vi "2 HeadingChooser.vi"() -> (2 "Optimal Heading Out":dbl, 3 "Goodness Functions":T3, 10 "Goodness Weightings":T2={"Target Importance"=0.98, "No Sail Importance"=1.0, "Change Importance"=0.2, "Pure Waypoint \nImportance"=0.0, "Pure Wind \nImportance"=0.0} {"Pure Wind \nImportance" min=0.0 step=0.2; "Pure Waypoint \nImportance" min=0.0 step=0.2; "Change Importance" min=0.0 step=0.2; "No Sail Importance" min=0.0 step=0.2; "Target Importance" min=0.0 step=0.2})   [LabVIEW 2011]
doc: "The Heading Chooser VI is responsible for finding the optimal heading for the boat in order to reach the waypoint. It uses fuzzy-logic inspired goodness function logic to choose a heading. Specifically, the VI takes 3 goodness function curves and makes a weighted combination of them, choosing the heading with the highest total goodness.\n\nThis VI does not contain any code that would limit the component goodness functions to just 3 or to the specific ones of 'target', 'no sail', and 'change'. Only the labels would need changing."
uses:
  2 Typedefs/Goodness Fns Indicator.ctl
  2 Typedefs/Goodness Weightings.ctl
  2 Classes/Waypoint/Waypoint.lvclass
  2 Globals/2 TuningConstants.vi
  2 Globals/2 Global.vi
panel:
  in  "Irons direct vector":T1 {"Origin"."North" format="%#_10f"; "Origin"."East" format="%#_8f"}
  out "start of wire":dbl
  out "end of wire":dbl
  # "huh???\nTODO: talk to NI about this"
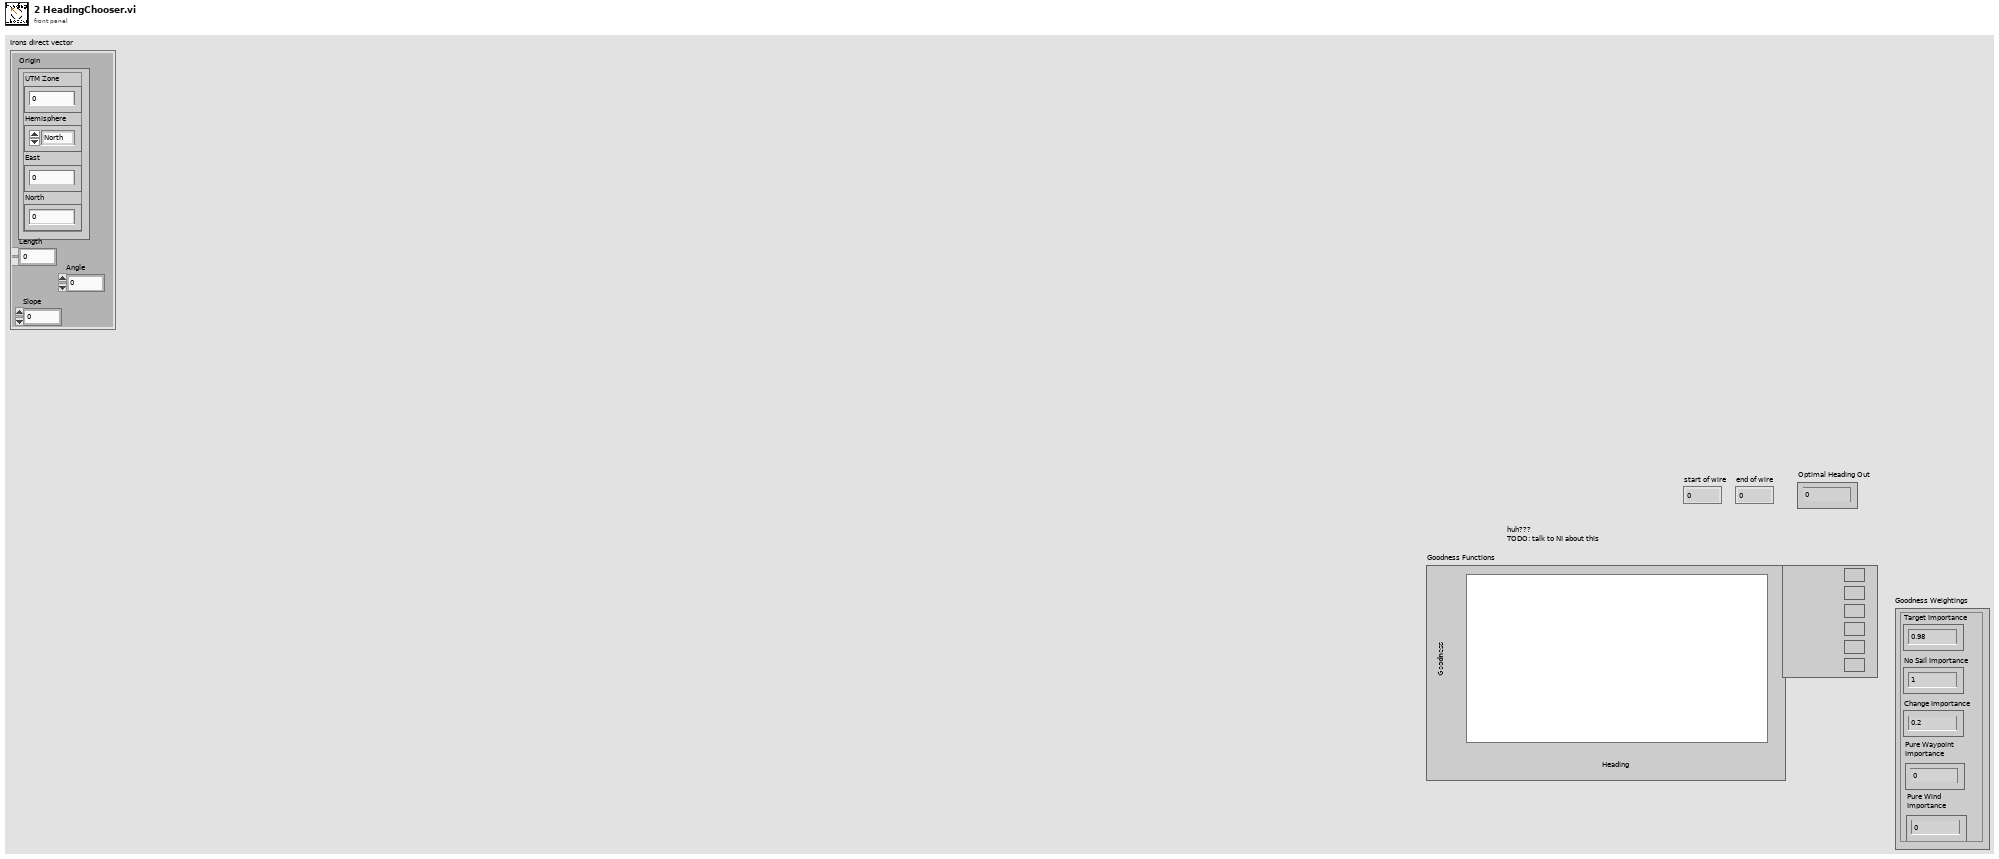
[diagram p1: front panel]
types:
  T1 = cluster{"Origin":cluster{"UTM Zone":dbl, "Hemisphere":enum16{"North", "South"}, "East":dbl, "North":dbl}, "Length":dbl, "Angle":dbl, "Slope":dbl}
  T2 = typedef "Goodness Weightings.ctl" = cluster{"Target Importance":dbl, "No Sail Importance":dbl, "Change Importance":dbl, "Pure Waypoint \nImportance":dbl, "Pure Wind \nImportance":dbl}
  T3 = typedef "Goodness Fns Indicator.ctl" = cluster{dbl, dbl, dbl[][]}
  T4 = typedef "UTM Location.ctl" = cluster{"UTM Zone":dbl, "Hemisphere":enum16{"North", "South"}, "East":dbl, "North":dbl}
  T5 = typedef "absolute wind direction.ctl" = dbl
  T6 = typedef "apparent wind direction.ctl" = dbl
  T7 = typedef "heading.ctl" = dbl
  T8 = cluster{"UTM Zone":dbl, "Hemisphere":enum16{"North", "South"}, "East":dbl, "North":dbl}
  T9 = cluster{"UTM Zone":bool, "Hemisphere":bool, "East":bool, "North":bool}
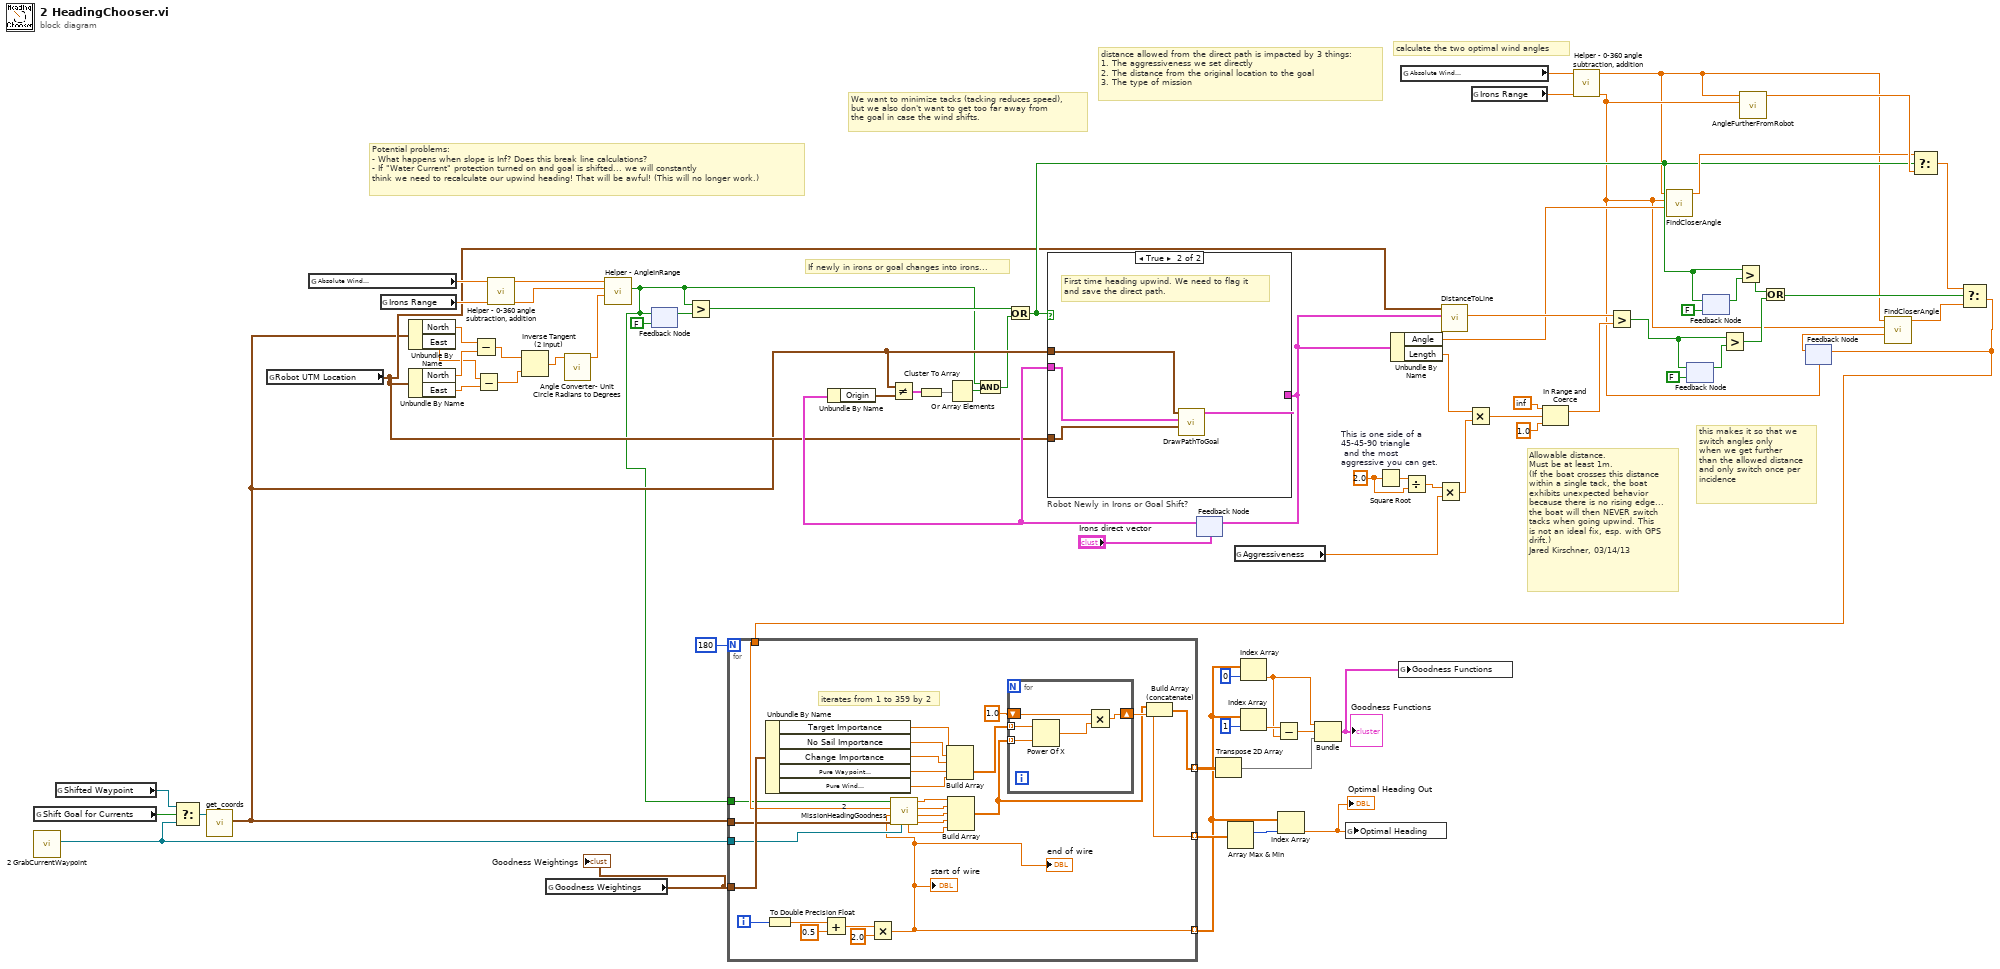
[diagram p0: block diagram]
diagram:
  w40 = 2.0 ("x")
  # "Potential problems:\n- What happens when slope is Inf? Does this break line calculations?\n- If \"Water Current\" protection turned on and goal is shifted... we will constantly\nthink we need to recalculate our upwind heading! That will be awful! (This will no longer work.)"
  # "If newly in irons or goal changes into irons..."
  # "Allowable distance.\nMust be at least 1m.\n(If the boat crosses this distance\nwithin a single tack, the boat\nexhibits unexpected behavior\nbecause there is no rising edge...\nthe boat will then NEVER switch\ntacks when going upwind. This\nis not an ideal fix, esp. with GPS\ndrift.)\nJared Kirschner, 03/14/13"
  # "this makes it so that we\nswitch angles only\nwhen we get further\nthan the allowed distance\nand only switch once per\nincidence"
  # "calculate the two optimal wind angles"
  # "distance allowed from the direct path is impacted by 3 things:\n1. The aggressiveness we set directly\n2. The distance from the original location to the goal\n3. The type of mission"
  # "We want to minimize tacks (tacking reduces speed),\nbut we also don't want to get too far away from\nthe goal in case the wind shifts."
  n1 = global read "2 Global.vi" "Shift Goal for Currents"() -> (w62:bool)
  n2 = call "2 GrabCurrentWaypoint.vi"() -> ("Current Waypoint"=w61:refnum<class "Waypoint.lvclass">)  [unwired: 11 in]
  n3 = global read "2 Global.vi" "Shifted Waypoint"() -> (w63:refnum<class "Waypoint.lvclass">)
  n4 = Select(t=w63, s=w62, f=w61) -> (s? t:f=w60:refnum<class "Waypoint.lvclass">)
  n5 = call-dynamic "get_coords.vi"("Waypoint in"=w60) -> ("Coords"=w17:T4)  [unwired: 7 in, 3 out]
  n6 = global read "2 Global.vi" "Robot UTM Location"() -> (w18:T4)
  n7 = global read "2 Global.vi" "Absolute Wind\nDirection (º)"() -> (w48:T5)
  n8 = global read "2 TuningConstants.vi" "Irons Range"() -> (w49:dbl)
  n9 = Unbundle By Name(w17) -> ("North"=w53:dbl, "East"=w51:dbl)
  n10 = Unbundle By Name(w18) -> ("North"=w52:dbl, "East"=w50:dbl)
  n11 = Subtract(x=w53, y=w52) -> (x-y=w56:dbl)
  n12 = Subtract(x=w51, y=w50) -> (x-y=w55:dbl)
  n13 = call "Helper - 0-360 angle subtraction, addition.vi"("y"=w49, "x"=w48) -> ("x + y"=w46:dbl, "x - y"=w47:T6)  [unwired: 8 in]
  n14 = Inverse Tangent (2 Input)(1:w55, 2:w56) -> (0:w54:dbl)
  n15 = global read "2 TuningConstants.vi" "Goodness Weightings"() -> (w69:T2)
  "Goodness Weightings" <- w69
  n16 = call "Angle Converter- Unit Circle Radians to Degrees.vi"("Angle in \nUnit Circle\nRadians"=w54) -> ("Angle in \nHeading \nFormat"=w57:T7)  [unwired: 10 in]
  n17 = call "Helper - AngleInRange.vi"("Angle to check"=w57, "Angle 2"=w46, "Angle 1"=w47) -> ("In range?"=w15:bool)  [unwired: 8 in]
  n18 = feedback-in #1(w15) -> ()
  n19 = feedback #1(FALSE ("In irons?")) -> (w44:bool)
  n20 = Greater?(x=w15, y=w44) -> (0:w28:bool)
  n21 = feedback #2("Irons direct vector") -> (w39:T1)
  n22 = Unbundle By Name(w39) -> ("Origin"=w38:T8)
  n23 = Not Equal?(x=w17, y=w38) -> (x != y?=w37:T9)
  n24 = Cluster To Array(cluster=w37) -> (array=w36:bool[])
  n25 = Or Array Elements(Boolean array=w36) -> (logical OR=w16:bool)
  n26 = And(x=w15, y=w16) -> (x .and. y?=w14:bool)
  n27 = Or(x=w28, y=w14) -> (x .or. y?=w20:bool)
  n28 = case "Robot Newly in Irons or Goal Shift?" shown="True" w20 {
    tunnel: w39 -> [w76 w80]
    tunnel: w17 -> [_ w79]
    tunnel: w18 -> [_ w78]
    tunnel: [w76 w77] -> w7
    frame False {
    }
    frame True {
      # "First time heading upwind. We need to flag it\nand save the direct path."
      n29 = call "DrawPathToGoal.vi"("Robot UTM Location"=w78, "Irons direct vector in"=w80, "Goal"=w79) -> ("Irons direct vector out"=w77:T1)  [unwired: 8 in]
    }
  }
  n30 = feedback-in #2(w7) -> ()
  n31 = global read "2 TuningConstants.vi" "Aggressiveness"() -> (w31:dbl)
  n32 = Square Root(x=w40) -> (sqrt(x)=w41:dbl)
  n33 = Unbundle By Name(w7) -> ("Angle"=w5:dbl, "Length"=w6:dbl)
  n34 = global read "2 Global.vi" "Absolute Wind\nDirection (º)"() -> (w34:T5)
  n35 = Divide "This is one side of a 45-45-90 triangle\n and the most aggressive you can get."(x=w41, y=w40) -> (x/y=w33:dbl)
  n36 = Multiply(x=w33, y=w31) -> (x*y=w32:dbl)
  n37 = call "DistanceToLine.vi"("Irons direct vector out"=w7, "Robot UTM Location"=w18) -> ("Distance"=w42:dbl)  [unwired: 9 in]
  n38 = Multiply(x=w6, y=w32) -> (x*y=w11:dbl)
  n39 = global read "2 TuningConstants.vi" "Irons Range"() -> (w35:dbl)
  n40 = In Range and Coerce(upper limit=inf, x=w11, lower limit=1.0) -> (coerced(x)=w10:dbl)  [unwired: 1 out]
  n41 = call "Helper - 0-360 angle subtraction, addition.vi"("y"=w35, "x"=w34) -> ("x + y"=w3:dbl, "x - y"=w2:T6)  [unwired: 8 in]
  n42 = Greater?(x=w42, y=w10) -> (0:w23:bool)
  n43 = call "FindCloserAngle.vi"("Central Angle"=w5, "Angle 2"=w3, "Angle 1"=w2) -> ("Closer Angle"=w26:T6)  [unwired: 8 in]
  n44 = feedback #3(FALSE) -> (w25:bool)
  n45 = feedback-in #3(w23) -> ()
  n46 = feedback #4(FALSE) -> (w21:bool)
  n47 = feedback-in #4(w20) -> ()
  n48 = Greater?(x=w23, y=w25) -> (0:w12:bool)
  n49 = Greater?(x=w20, y=w21) -> (0:w13:bool)
  n50 = call "AngleFurtherFromRobot.vi"("Angle 2"=w3, "Angle 1"=w2) -> ("Angle further from Robot"=w27:T6)  [unwired: 9 in]
  n51 = Or(x=w13, y=w12) -> (x .or. y?=w19:bool)
  n52 = feedback #5(w3) -> (w4:T6)
  n53 = call "FindCloserAngle.vi"("Central Angle"=w4, "Angle 2"=w3, "Angle 1"=w2) -> ("Closer Angle"=w1:T6)  [unwired: 8 in]
  n54 = Select(t=w26, s=w20, f=w27) -> (s? t:f=w30:T6)
  n55 = Select(t=w30, s=w19, f=w1) -> (s? t:f=w29:T6)
  n56 = for {
    N: 180 -> [_]
    tunnel: [w101] -> w67 mode=indexing
    tunnel: w69 -> [w105]
    tunnel: w61 -> [w104]
    tunnel: w17 -> [w103]
    tunnel: [w102] -> w68 mode=indexing
    tunnel: [w93] -> w59 mode=indexing
    tunnel: w29 -> [w82]
    tunnel: w15 -> [w81]
    i -> [w106]
    # "iterates from 1 to 359 by 2"
    n57 = Unbundle By Name(w105) -> ("Target Importance"=w88:dbl, "No Sail Importance"=w89:dbl, "Change Importance"=w90:dbl, "Pure Waypoint \nImportance"=w91:dbl, "Pure Wind \nImportance"=w92:dbl)
    n58 = To Double Precision Float(number=w106) -> (double precision float=w99:dbl)
    n59 = Add(x=w99, y=0.5) -> (x+y=w98:dbl)
    n60 = Multiply(x=w98, y=2.0) -> (x*y=w93:dbl)
    "end of wire" <- w93
    "start of wire" <- w93
    n61 = call "2 MissionHeadingGoodness.vi"("Waypoint in"=w104, "Waypoint Location"=w103, "Heading\nto Test"=w93, "UW Tack"=w82, "Into irons?"=w81) -> ("Pure Waypoint Goodness"=w84:dbl, "Direction Change Goodness"=w85:dbl, "No-Sail Goodness"=w86:dbl, "Target Goodness"=w87:dbl, "Pure Wind Goodness"=w83:dbl)  [unwired: 2 in]
    n62 = Build Array(w88, w89, w90, w91, w92) -> (w95:dbl[])
    n63 = Build Array(w87, w86, w85, w84, w83) -> (w94:dbl[])
    n64 = for {
      tunnel: w94 -> [w111] mode=indexing
      tunnel: w95 -> [w110] mode=indexing
      shift-right: [w108] -> w101
      shift-left: 1.0 -> [w107]
      n65 = Power Of X(1:w111, 2:w110) -> (0:w109:dbl)
      n66 = Multiply(x=w107, y=w109) -> (x*y=w108:dbl)
    }
    n67 = Build Array (concatenate)(w94, w101) -> (w102:dbl[])
  }
  n68 = Transpose 2D Array(2D array=w68) -> (transposed array=w64:dbl[][])
  n69 = Array Max & Min(array=w67) -> (max index (indices)=w71:i32)  [unwired: 3 out]
  n70 = Index Array(array=w59, index=0) -> (element=w66:dbl)
  n71 = Index Array(array=w59, index=1) -> (element=w74:dbl)
  n72 = Subtract(x=w74, y=w66) -> (x-y=w65:dbl)
  n73 = Index Array(array=w59, index=w71) -> (element=w58:dbl)
  "Optimal Heading Out" <- w58
  n74 = Bundle(w66, w65, w64) -> (w70:cluster{dbl, dbl, dbl[][]})  [unwired: 1 in]
  "Goodness Functions" <- w70
  n75 = global write "2 Global.vi" "Optimal Heading"(w58) -> ()
  n76 = global write "2 Global.vi" "Goodness Functions"(w70) -> ()
  n77 = feedback-in #5(w29) -> ()
